vi "Agilent6680AControl.vi"(9 "Function":u16(ring) items=["连接", "输出电流", "停止输出", "断开连接"], 10 "Curr1":dbl=40.0, 11 "6680A Port":string="*rst") -> (3 "result":i32)   [LabVIEW 2013]
panel:
  in  "控制读取  2":bool
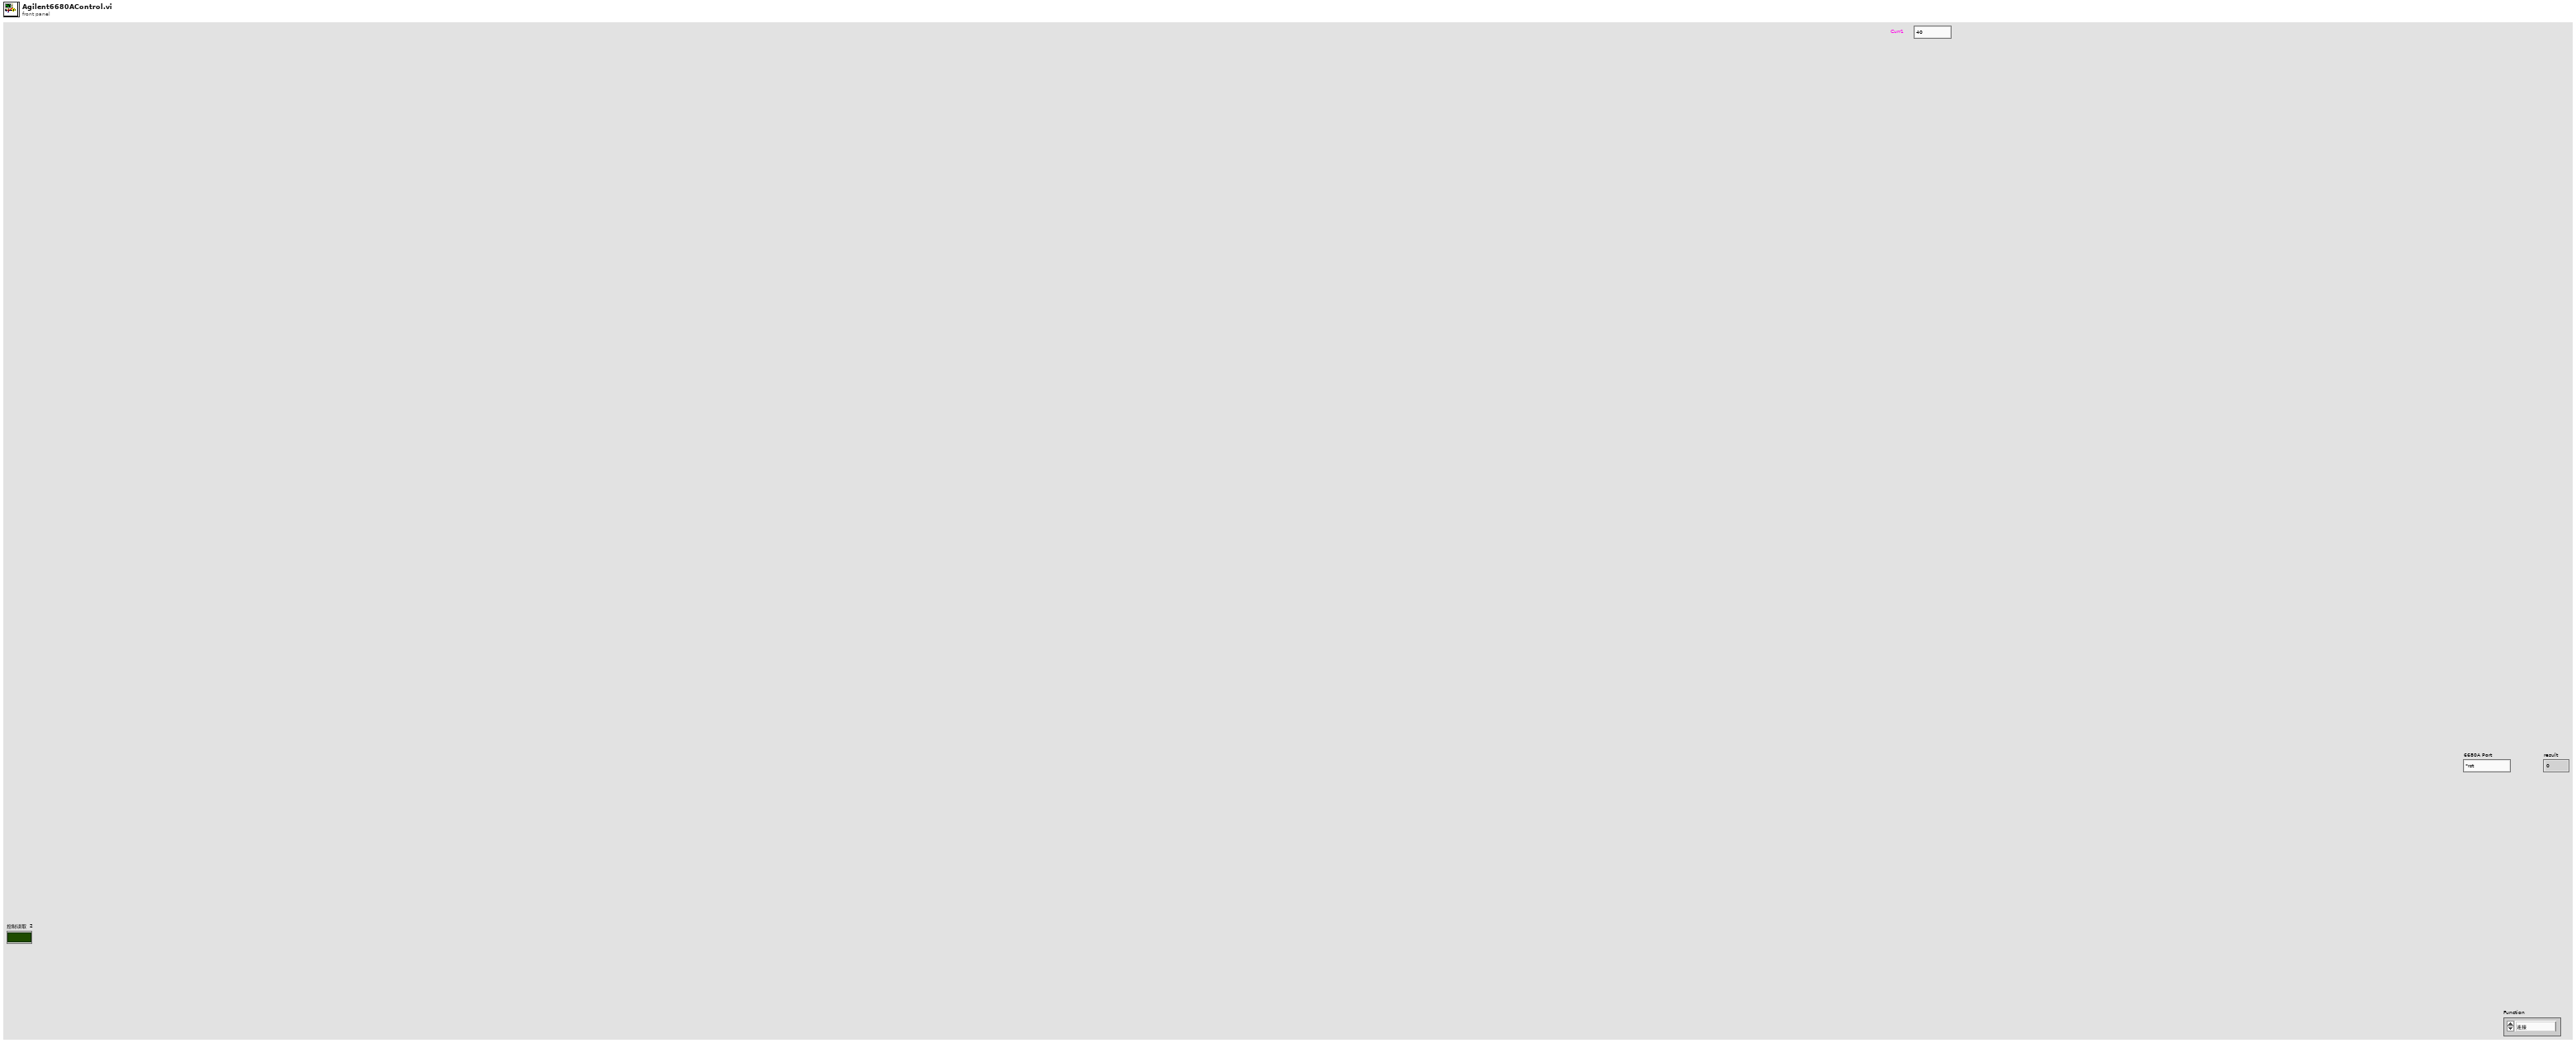
[diagram p1: front panel]
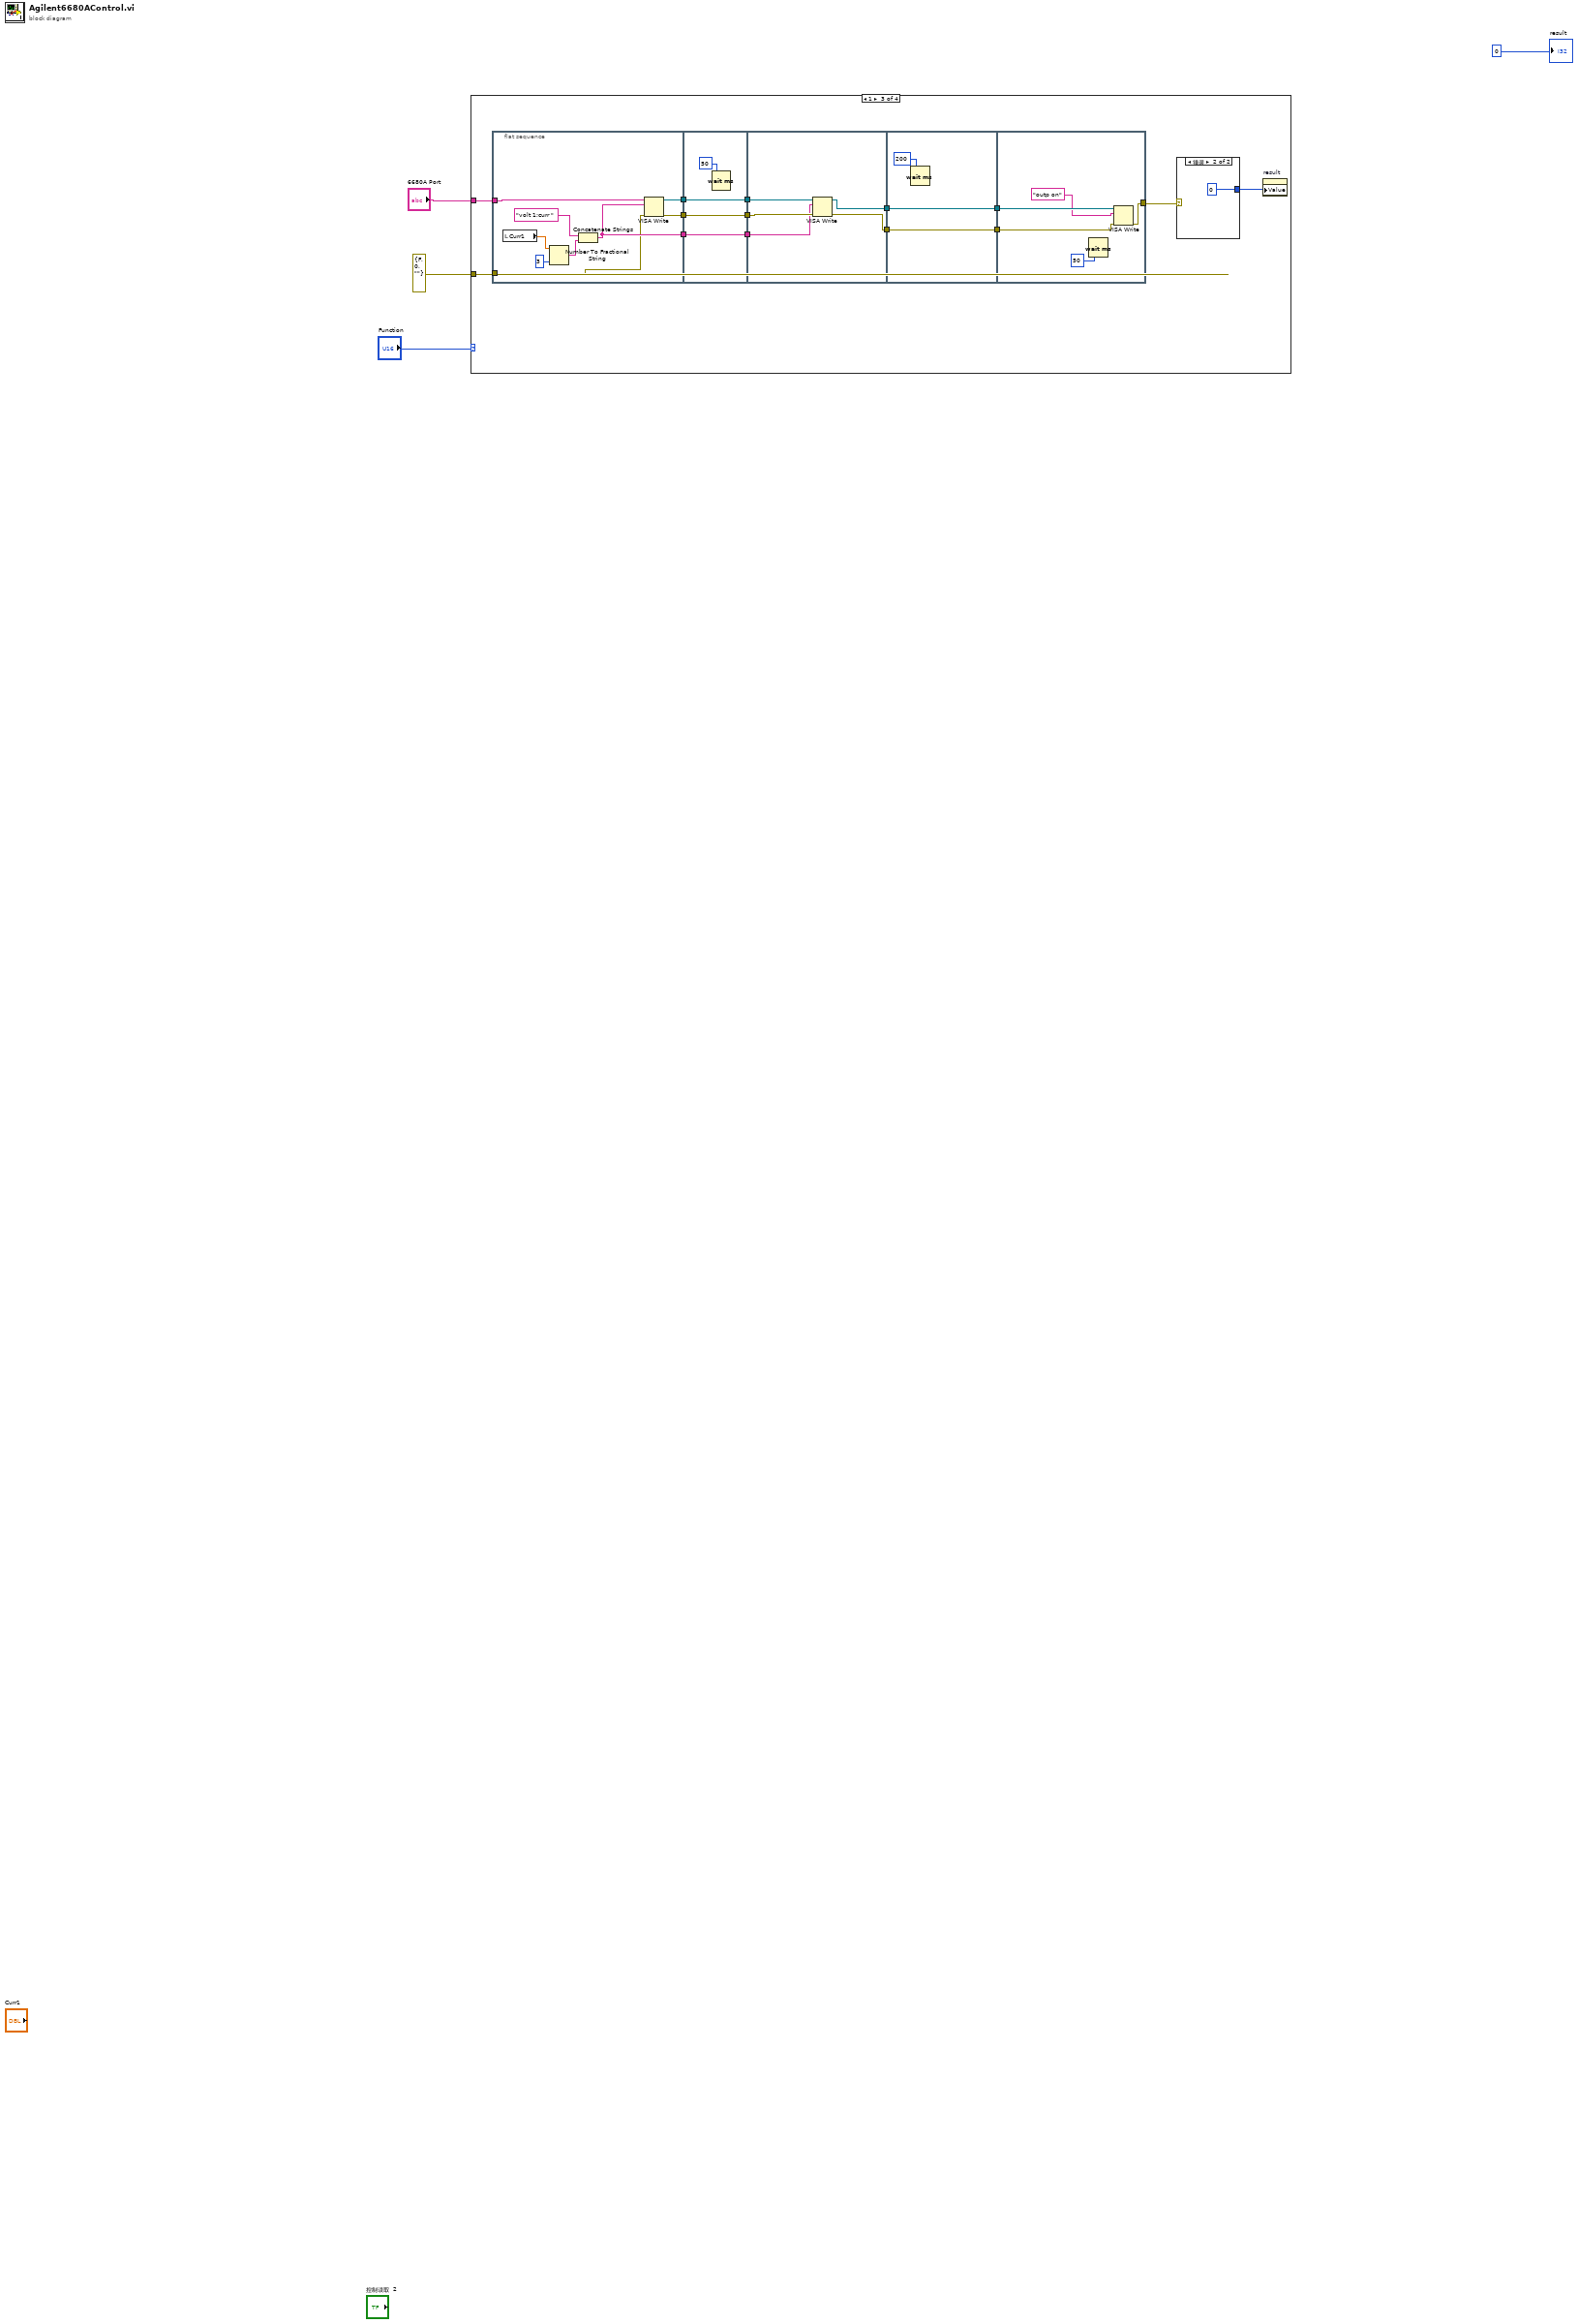
[diagram p0: block diagram]
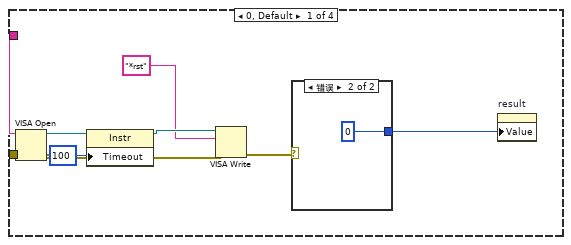
[diagram p2: hidden frame]
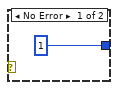
[diagram p3: hidden frame]
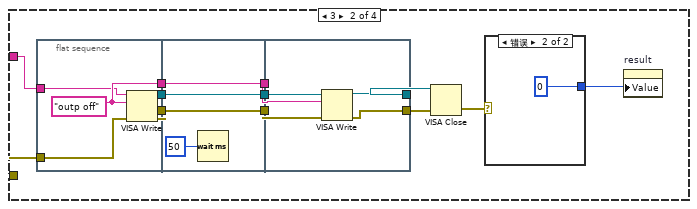
[diagram p4: hidden frame]
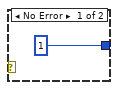
[diagram p5: hidden frame]
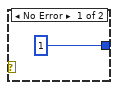
[diagram p6: hidden frame]
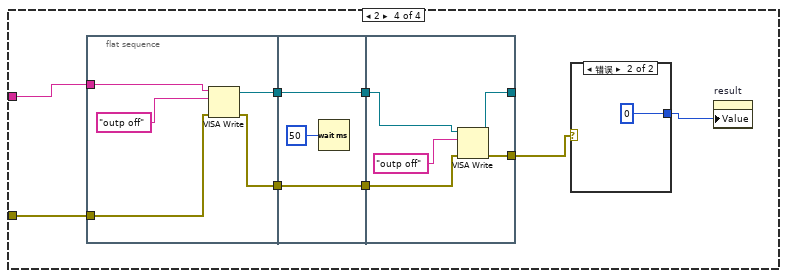
[diagram p7: hidden frame]
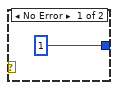
[diagram p8: hidden frame]
diagram:
  n1 = case shown="1" "Function" {
    tunnel: errorcluster {"status"=FALSE, "code"=0, "source"=""} ("错误输入（无错误）") -> [w9 w25 w46 w88]
    tunnel: "6680A Port" -> [w5 w24 w47 w89]
    frame 0, Default {
      n2 = VISA Open(error in (no error)=w9, VISA resource name=w5) -> (VISA resource name=w11:refnum<visa-resource-name>, error out=w13:errorcluster)  [unwired: 3 out]
      n3 = property class="Instr"(reference=w11, "Timeout"=u32 100 ("General Settings:Timeout Value")) -> (reference out=w10:refnum<visa-resource-name>)  [unwired: 1 in, 1 out]
      n4 = VISA Write(VISA resource name=w10, write buffer="*rst" ("写入缓冲区"), error in (no error)=w13) -> (error out=w7:errorcluster)  [unwired: 2 out]
      n5 = case shown="错误" w7 {
        tunnel: [1 0] -> w6
        frame No Error {
        }
        frame Error {
        }
      }
      n6 = property on="result" class="DigNum (严格)"("Value"=w6) -> ()  [unwired: 2 in, 2 out]
    }
    frame 3 {
      n7 = flat-sequence {
        tunnel: [w34] -> w23
        tunnel: [w33] -> w21
        tunnel: [w32] -> w19
        tunnel: w24 -> [w30]
        tunnel: w25 -> [w31]
        tunnel: w23 -> [w38]
        tunnel: [w38] -> w22
        tunnel: w21 -> [w37]
        tunnel: [w37] -> w20
        tunnel: w19 -> [w36]
        tunnel: [w36] -> w18
        tunnel: [w41] -> w27
        tunnel: [w40] -> w26
        tunnel: w22 -> [w43]
        tunnel: w20 -> [w42]
        tunnel: w18 -> [w39]
        frame #0 {
          w32 = "outp off" ("写入缓冲区")
          n8 = VISA Write(VISA resource name=w30, write buffer=w32, error in (no error)=w31) -> (VISA resource name out=w34:refnum<visa-resource-name>, error out=w33:errorcluster)  [unwired: 1 out]
        }
        frame #1 {
          n9 = Wait (ms)(milliseconds to wait=u32 50 ("等待时间（毫秒）")) -> ()  [unwired: 1 out]
        }
        frame #2 {
          n10 = VISA Write(VISA resource name=w43, write buffer=w39, error in (no error)=w42) -> (VISA resource name out=w40:refnum<visa-resource-name>, error out=w41:errorcluster)  [unwired: 1 out]
        }
      }
      n11 = VISA Close(VISA resource name=w26, error in (no error)=w27) -> (error out=w16:errorcluster)
      n12 = case shown="错误" w16 {
        tunnel: [1 0] -> w17
        frame No Error {
        }
        frame Error {
        }
      }
      n13 = property on="result" class="DigNum (严格)"("Value"=w17) -> ()  [unwired: 2 in, 2 out]
    }
    frame 1 {
      n14 = flat-sequence {
        tunnel: [w68] -> w57
        tunnel: [w67] -> w56
        tunnel: [w62] -> w55
        tunnel: w47 -> [w61]
        tunnel: w46 -> [w60]
        tunnel: w57 -> [w72]
        tunnel: [w72] -> w54
        tunnel: w56 -> [w71]
        tunnel: [w71] -> w53
        tunnel: [w69] -> w52
        tunnel: w55 -> [w69]
        tunnel: w54 -> [w77]
        tunnel: w53 -> [w76]
        tunnel: [w75] -> w51
        tunnel: [w74] -> w50
        tunnel: w52 -> [w73]
        tunnel: w51 -> [w80]
        tunnel: [w80] -> w49
        tunnel: w50 -> [w79]
        tunnel: [w79] -> w48
        tunnel: w49 -> [w84]
        tunnel: w48 -> [w83]
        tunnel: [w81] -> w44
        frame #0 {
          n15 = local read "Curr1"() -> (w65:dbl)
          n16 = Number To Fractional String(number=w65, precision (6)=i16 3 ("精度(6)")) -> (F-format string=w63:string)  [unwired: 2 out]
          n17 = Concatenate Strings("volt 1;curr " ("写入缓冲区"), w63) -> (w62:string)
          n18 = VISA Write(VISA resource name=w61, write buffer=w62, error in (no error)=w60) -> (VISA resource name out=w68:refnum<visa-resource-name>, error out=w67:errorcluster)  [unwired: 1 out]
        }
        frame #1 {
          n19 = Wait (ms)(milliseconds to wait=u32 50 ("等待时间（毫秒）")) -> ()  [unwired: 1 out]
        }
        frame #2 {
          n20 = VISA Write(VISA resource name=w77, write buffer=w73, error in (no error)=w76) -> (VISA resource name out=w75:refnum<visa-resource-name>, error out=w74:errorcluster)  [unwired: 1 out]
        }
        frame #3 {
          n21 = Wait (ms)(milliseconds to wait=u32 200 ("等待时间（毫秒）")) -> ()  [unwired: 1 out]
        }
        frame #4 {
          n22 = Wait (ms)(milliseconds to wait=u32 50 ("等待时间（毫秒）")) -> ()  [unwired: 1 out]
          n23 = VISA Write(VISA resource name=w84, write buffer="outp on" ("写入缓冲区"), error in (no error)=w83) -> (error out=w81:errorcluster)  [unwired: 2 out]
        }
      }
      n24 = case shown="错误" w44 {
        tunnel: [1 0] -> w45
        frame No Error {
        }
        frame Error {
        }
      }
      n25 = property on="result" class="DigNum (严格)"("Value"=w45) -> ()  [unwired: 2 in, 2 out]
    }
    frame 2 {
      n26 = flat-sequence {
        tunnel: [w98] -> w93
        tunnel: [w97] -> w92
        tunnel: w89 -> [w99]
        tunnel: w88 -> [w96]
        tunnel: w93 -> [w103]
        tunnel: [w103] -> w91
        tunnel: [w101] -> w90
        tunnel: w92 -> [w101]
        tunnel: [w106] -> _
        tunnel: w91 -> [w107]
        tunnel: w90 -> [w105]
        tunnel: [w104] -> w87
        frame #0 {
          n27 = VISA Write(VISA resource name=w99, write buffer="outp off" ("写入缓冲区"), error in (no error)=w96) -> (VISA resource name out=w98:refnum<visa-resource-name>, error out=w97:errorcluster)  [unwired: 1 out]
        }
        frame #1 {
          n28 = Wait (ms)(milliseconds to wait=u32 50 ("等待时间（毫秒）")) -> ()  [unwired: 1 out]
        }
        frame #2 {
          n29 = VISA Write(VISA resource name=w107, write buffer="outp off" ("写入缓冲区"), error in (no error)=w105) -> (VISA resource name out=w106:refnum<visa-resource-name>, error out=w104:errorcluster)  [unwired: 1 out]
        }
      }
      n30 = case shown="错误" w87 {
        tunnel: [1 0] -> w86
        frame No Error {
        }
        frame Error {
        }
      }
      n31 = property on="result" class="DigNum (严格)"("Value"=w86) -> ()  [unwired: 2 in, 2 out]
    }
  }
  "result" <- 0
